vi "Day2_SerialRead.vi"() -> ()   [LabVIEW 2025]
uses:
  <vilib>/Utility/error.llb/Trim Whitespace One-Sided.vi
  <vilib>/Instr/_visa.llb/VISA Configure Serial Port (Instr).vi
panel:
  in  "stop":bool
  out "ADC (mv)":dbl
  out "Touch Pin":dbl
  out "Hall Sensor":dbl
  out "Timestamp":dbl
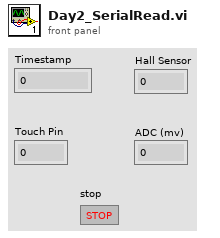
[diagram p1: front panel]
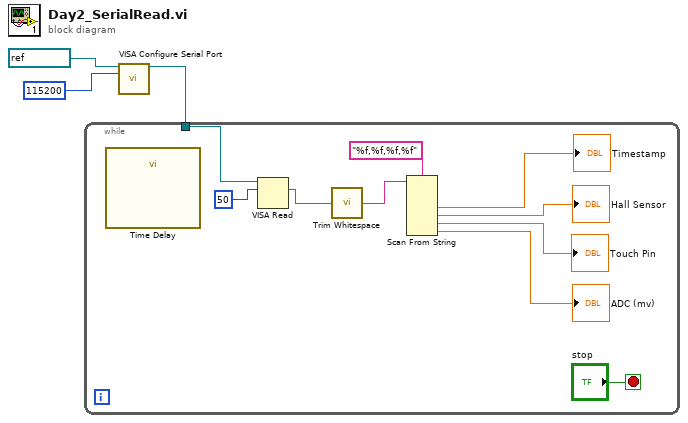
[diagram p0: block diagram]
diagram:
  n1 = call-poly "VISA Configure Serial Port"("VISA resource name"=refnum<visa-resource-name> "COM3", "baud rate (9600)"=u32 115200) -> ("VISA resource name out"=w2:refnum<visa-resource-name>)  [unwired: 12 in, 1 out]
  n2 = while {
    tunnel: w2 -> [w12]
    stop <- "stop" stop-if-true
    n3 = call "Time Delay"() -> ()  [unwired: 11 in, 1 out]
    n4 = VISA Read(VISA resource name=w12, byte count=u32 50) -> (read buffer=w10:string)  [unwired: 1 in, 3 out]
    n5 = call <vilib>:"Trim Whitespace.vi"("string"=w10) -> ("trimmed string"=w9:string)  [unwired: 1 in]
    n6 = Scan From String "Scan From String"(format string="%f,%f,%f,%f", input string=w9) -> (output 1=→"Timestamp":dbl, output 2=→"Hall Sensor":dbl, output 3=→"Touch Pin":dbl, output 4=→"ADC (mv)":dbl)  [unwired: 6 in, 3 out]
  }
